vi "rot.vi"(9 "angle":dbl, 10 "y":i32, 11 "x":i32) -> (2 "y'":i32, 3 "x'":i32)   [LabVIEW 2014]
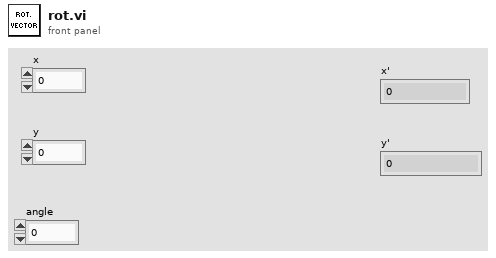
[diagram p1: front panel]
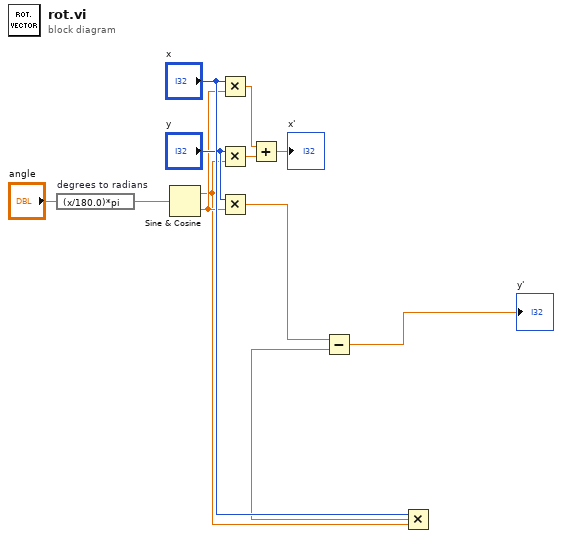
[diagram p0: block diagram]
diagram:
  n1 = expression code="(x/180.0)*pi" "degrees to radians"("angle") -> (w1:dbl)
  n2 = Sine & Cosine(0:w1) -> (1:w9:dbl, 2:w10:dbl)
  n3 = Multiply(x="x", y=w10) -> (x*y=w8:dbl)
  n4 = Multiply(x="y", y=w9) -> (x*y=w7:dbl)
  n5 = Multiply(x="y", y=w10) -> (x*y=w5:dbl)
  n6 = Add(x=w8, y=w7) -> (x+y=→"x'":dbl)
  n7 = Multiply(x="x", y=w9) -> (x*y=w4:dbl)
  n8 = Subtract(x=w5, y=w4) -> (x-y=→"y'":dbl)
